vi "CmdCenter_SingleRecipe.vi"(8 "error in (no error)":errorcluster, 11 "Message_Queues":T2) -> (0 "error out":errorcluster)   [LabVIEW 2014]
uses:
  15_DataManagement/Config_RFSG.ctl
  02_Controls/Message_Queues.ctl
  02_Controls/Message_Data_Ctl.ctl
  15_DataManagement/Config_RFSA_IQ_Acq.ctl
  15_DataManagement/Config_RFSA_Spectrum_Acq.ctl
  15_DataManagement/Config_RFSA_Vertical.ctl
  <vilib>/Utility/file.llb/Read From Spreadsheet File (string).vi
panel:
  in  "Recipe_Index":i32
  in  "file path (dialog if empty)":path=path "C:/Gyuwon_Folder/SourceCodeFolder/1005_Gyu_RF_SourceProject_Msg/___SystemFiles/RecipeMode.ini"
  in  "Tab Control":enum32{"RFSG_Config"}(tab)
  out "Config_RFSG":T1={"Carrier Frequency"=1300000000.0, "RF Power Level (dBm)"=-20.0, "SG External Gain (dBm)"=0.0, "Standard"=enum."LTE"} {"SG External Gain (dBm)" format="%#_6p"; "RF Power Level (dBm)" format="%#_6p"; "Carrier Frequency" format="%#_6p"}
  in  "Update":bool
  in  "Stop Button":bool
  in  "Start":bool
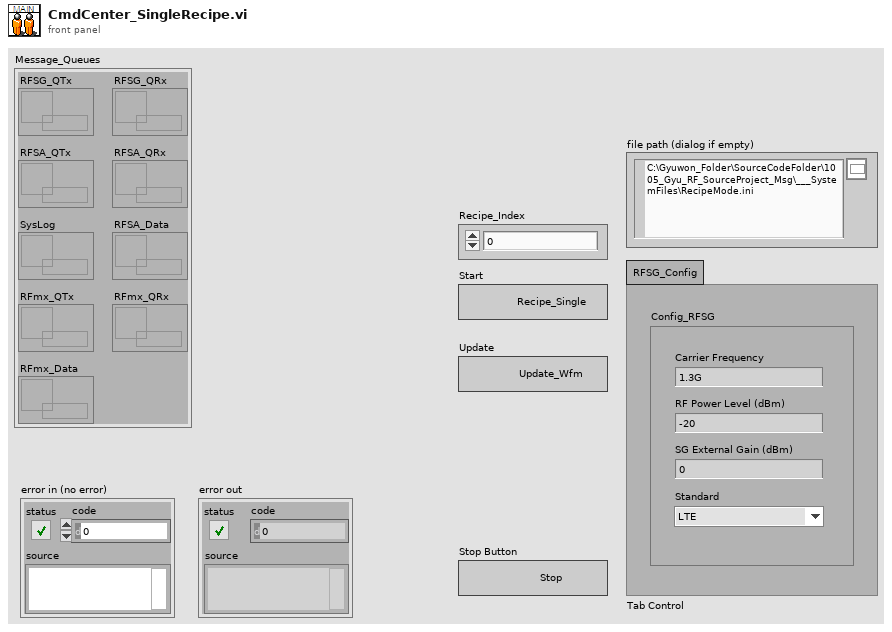
[diagram p1: front panel]
types:
  T1 = typedef "Config_RFSG.ctl" = cluster{"Carrier Frequency":dbl, "RF Power Level (dBm)":dbl, "SG External Gain (dBm)":dbl, "Standard":enum16{"LTE", "WCDMA", "GSM", "EDGE", "CW", "CWM"}}
  T2 = typedef "Message_Queues.ctl" = cluster{"RFSG_QTx":refnum<queue>, "RFSG_QRx":refnum<queue>, "RFSA_QTx":refnum<queue>, "RFSA_QRx":refnum<queue>, "SysLog":refnum<queue>, "RFSA_Data":refnum<queue>, "RFmx_QTx":refnum<queue>, "RFmx_QRx":refnum<queue>, "RFmx_Data":refnum<queue>}
  T3 = typedef "Config_RFSA_Vertical.ctl" = cluster{"Acquisition Type":i32, "Reference Level (dBm)":dbl, "External Gain (dB)":dbl}
  T4 = typedef "Config_RFSA_Spectrum_Acq.ctl" = cluster{"Resolution Bandwidth (Hz)":dbl, "Start Frequency (Hz)":dbl, "Stop Frequency (Hz)":dbl}
  T5 = typedef "Config_RFSA_IQ_Acq.ctl" = cluster{"carrier frequency":dbl, "IQ rate (S/s)":dbl, "samples per record":i64}
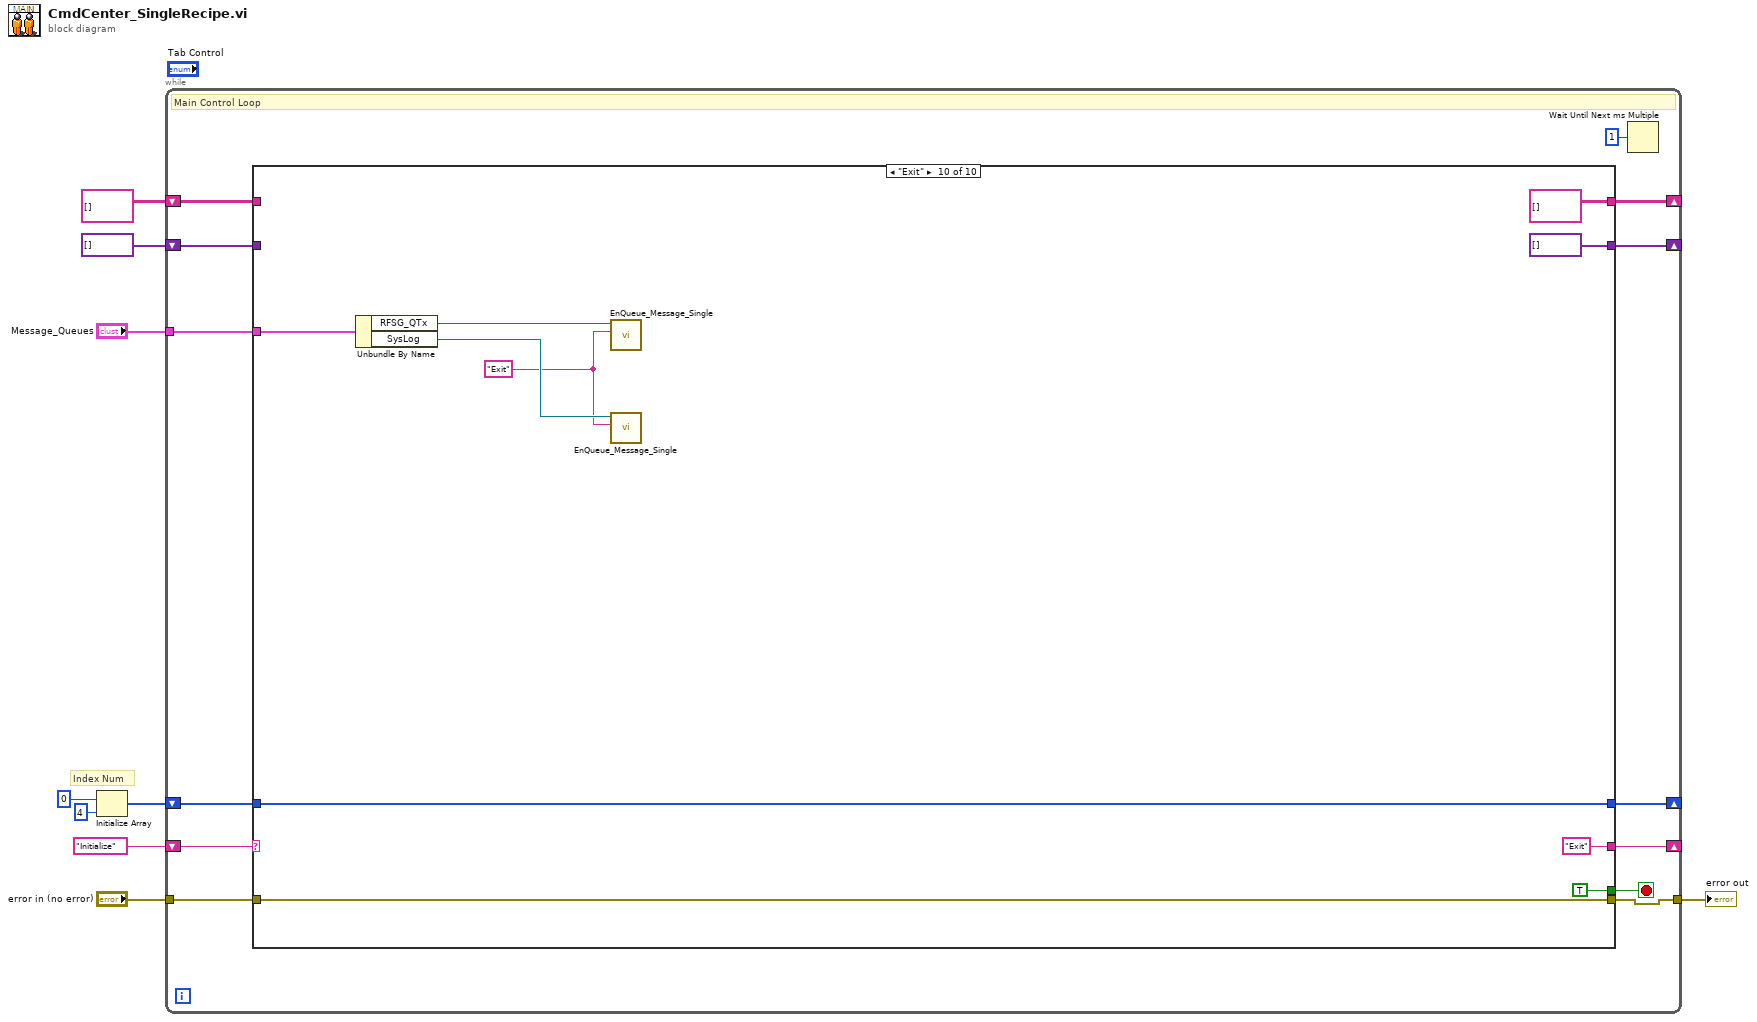
[diagram p0: block diagram]
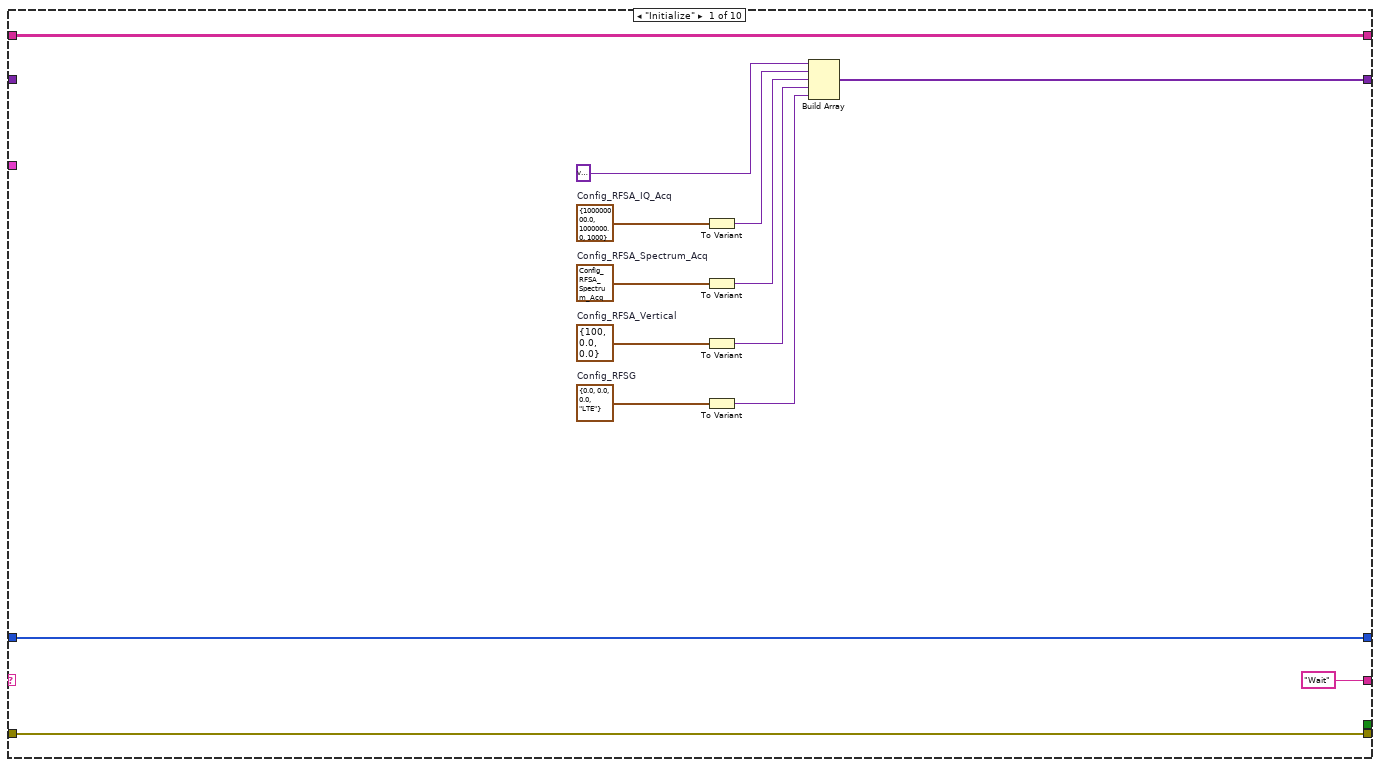
[diagram p2: hidden frame]
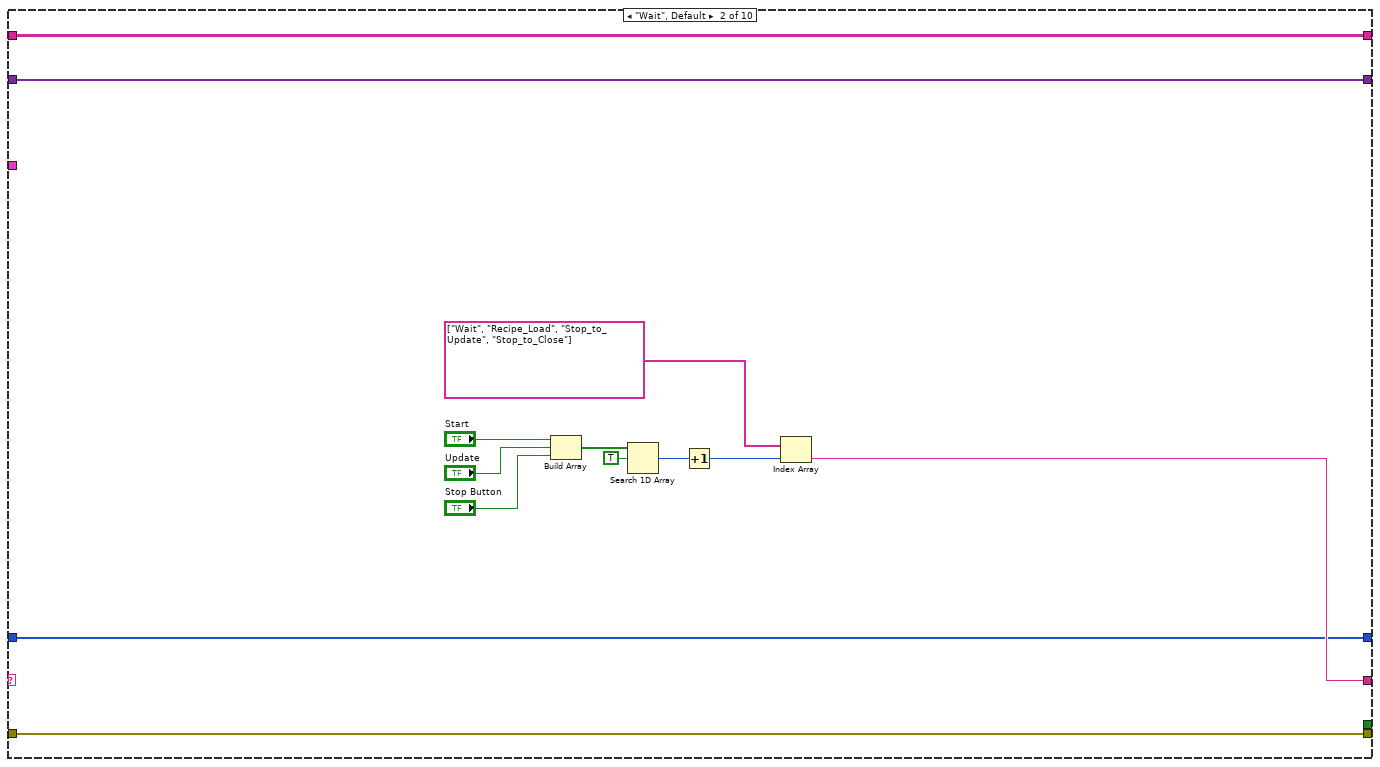
[diagram p3: hidden frame]
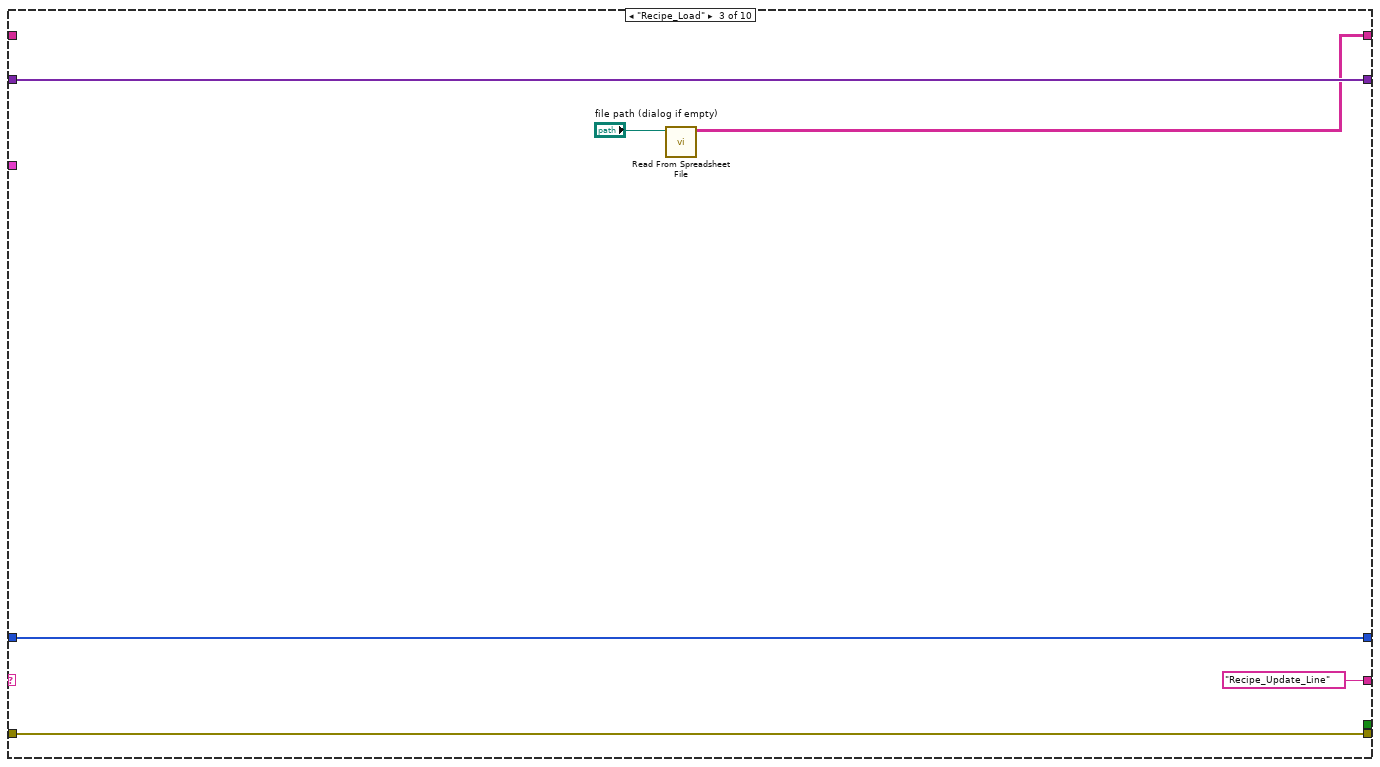
[diagram p4: hidden frame]
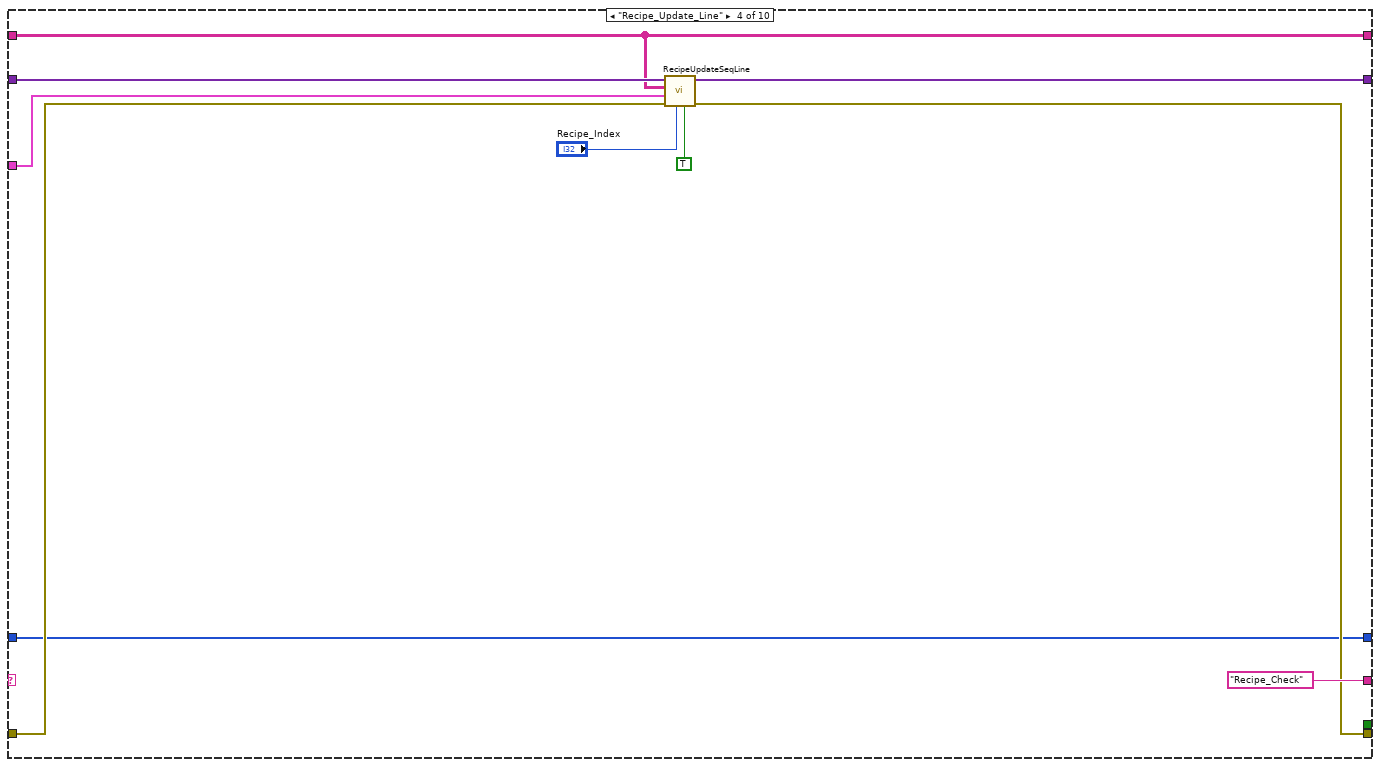
[diagram p5: hidden frame]
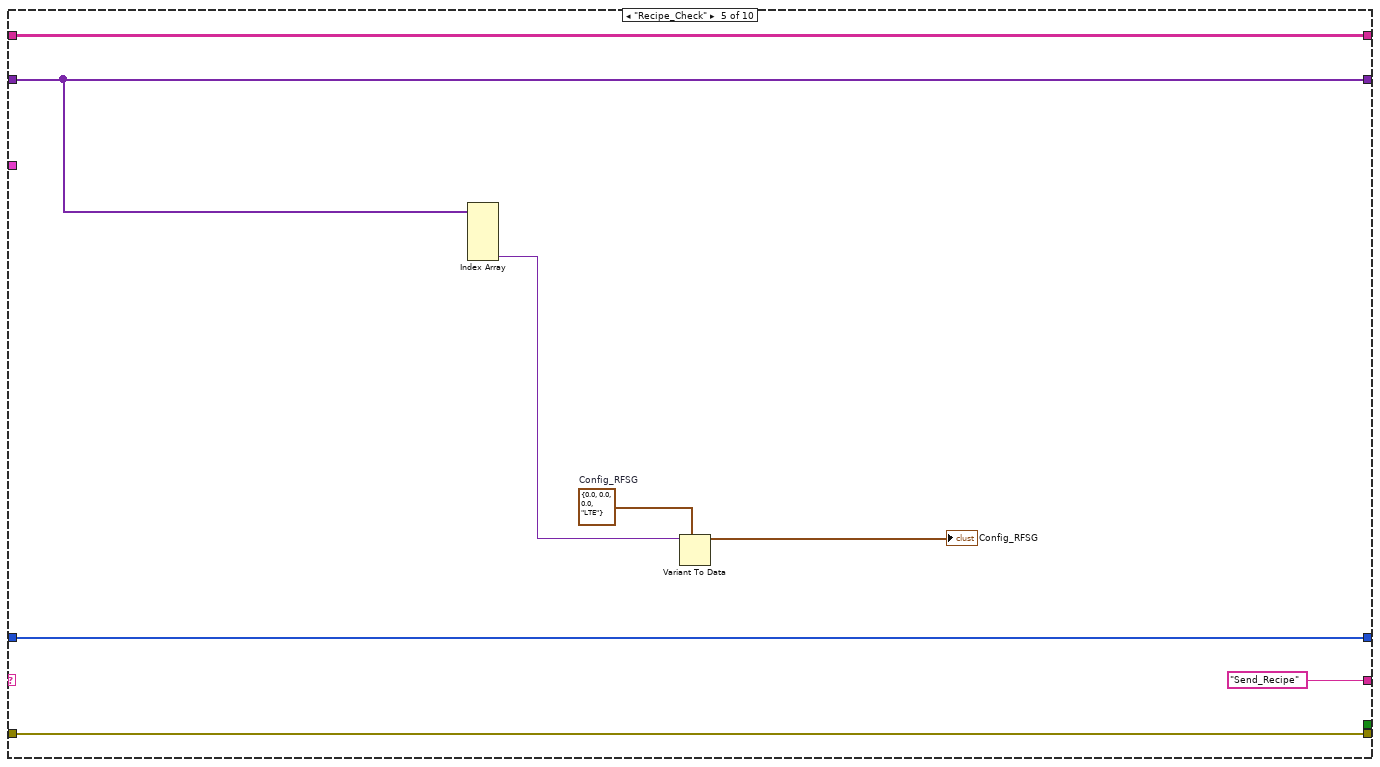
[diagram p6: hidden frame]
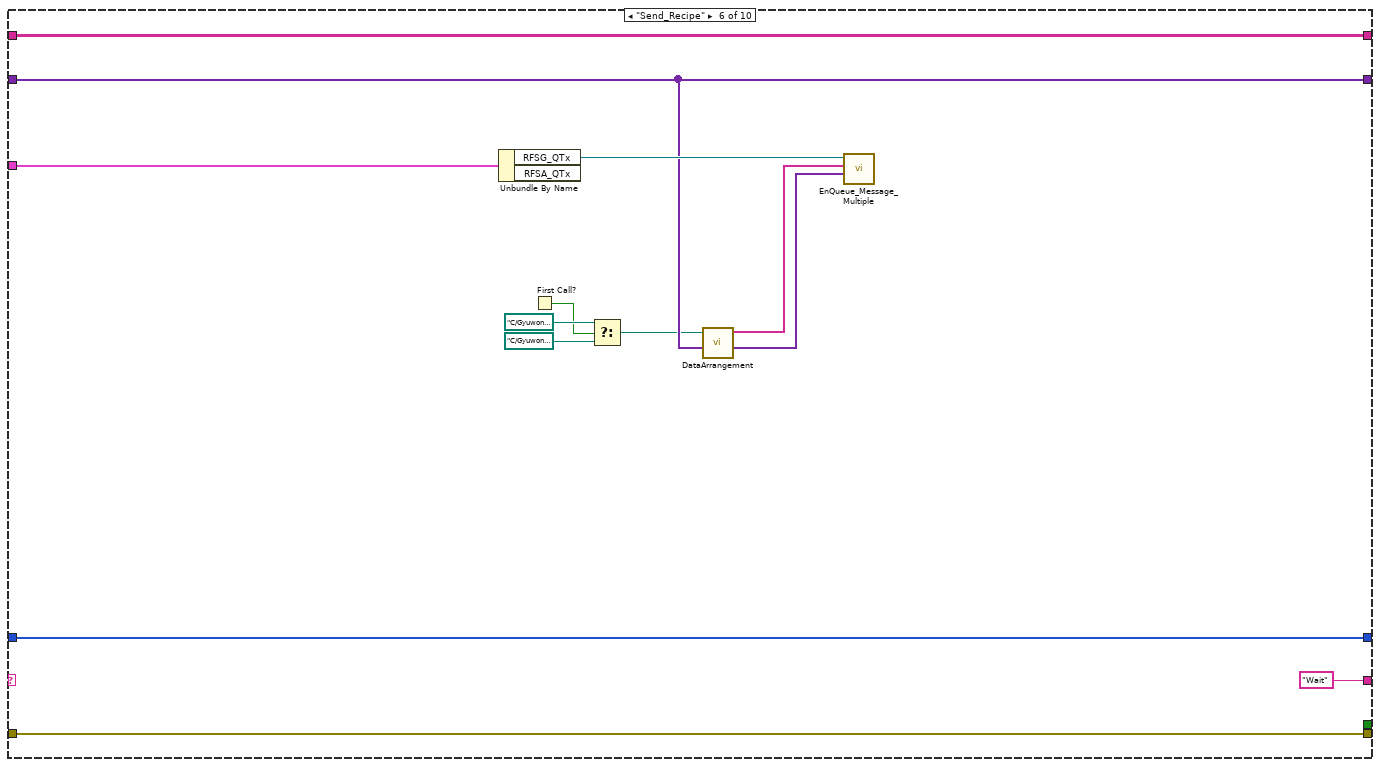
[diagram p7: hidden frame]
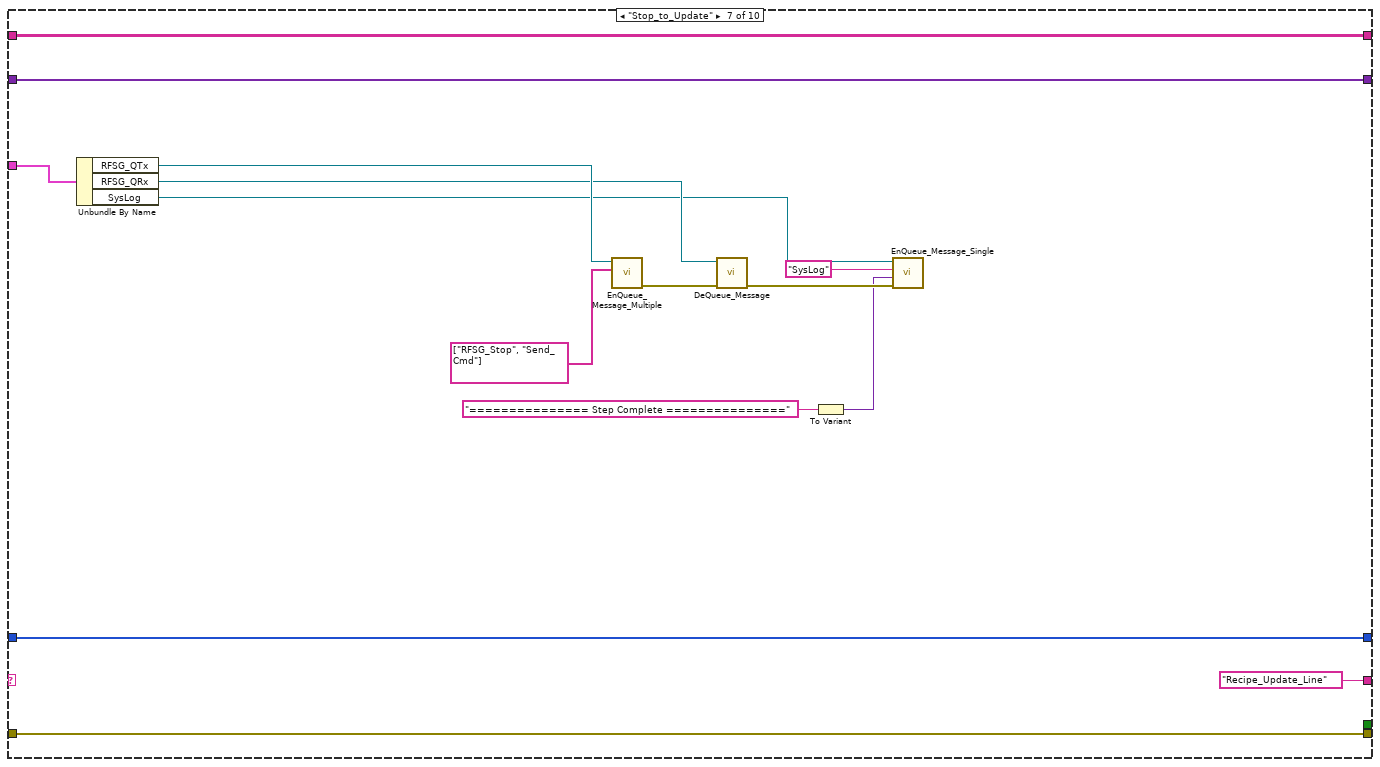
[diagram p8: hidden frame]
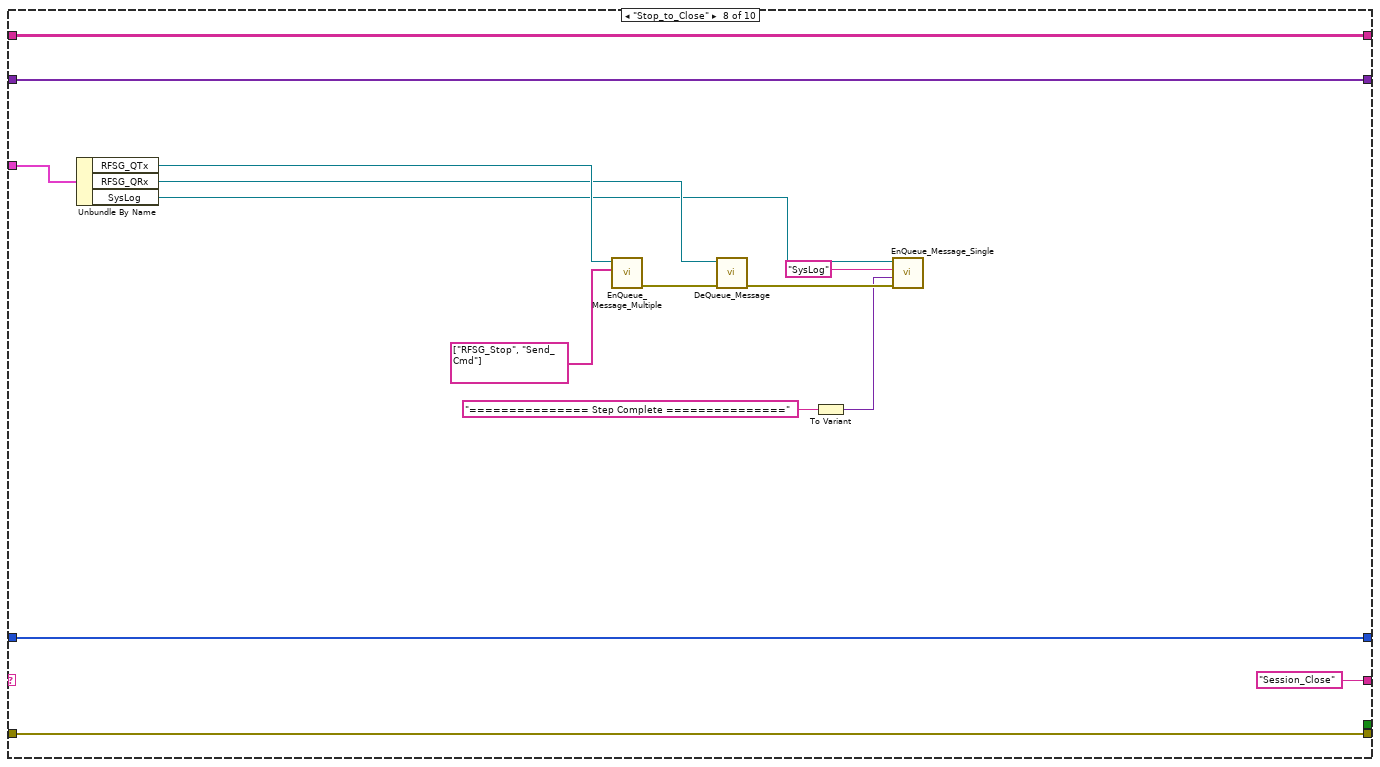
[diagram p9: hidden frame]
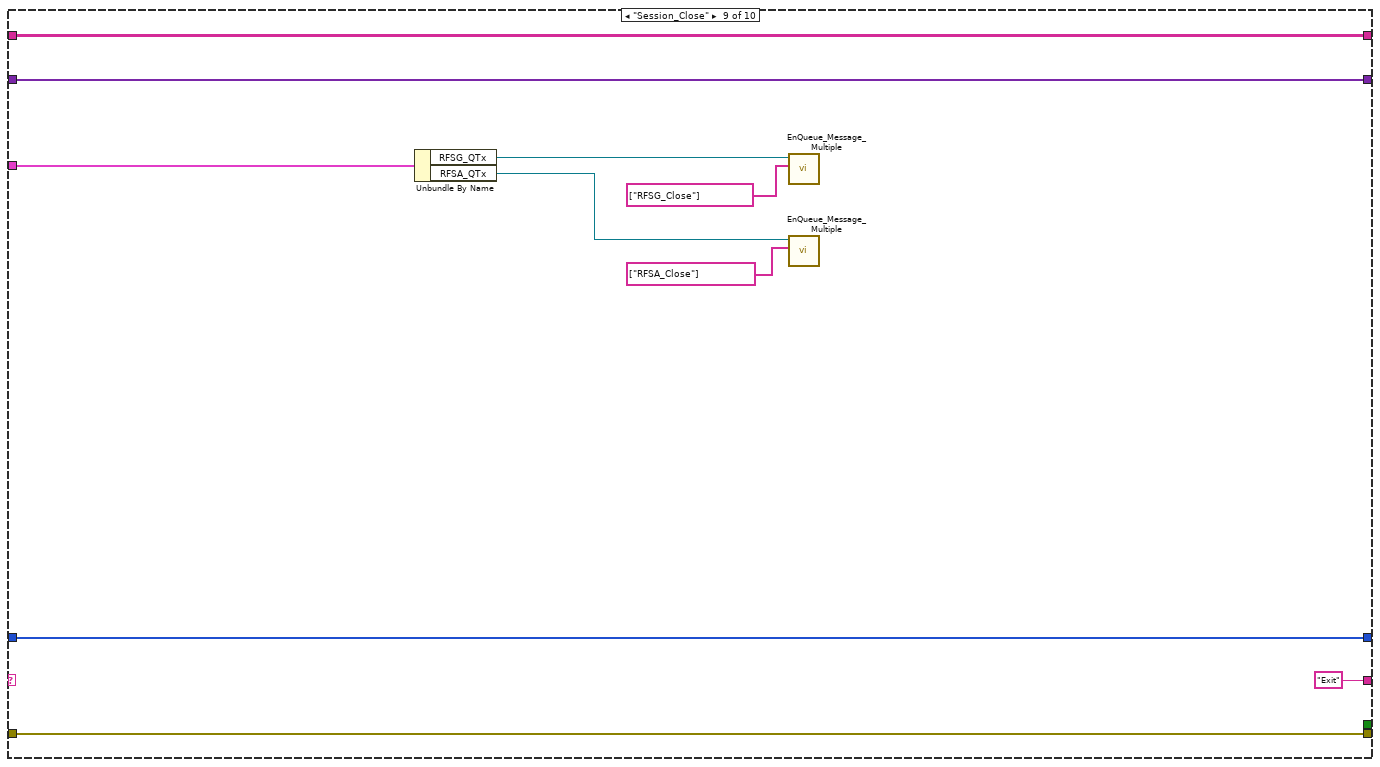
[diagram p10: hidden frame]
diagram:
  # "Index Num"
  n1 = Initialize Array(0, 4 ("dimension size")) -> (w1:i32[])
  n2 = while {
    tunnel: "error in (no error)" -> [w18]
    tunnel: [w21] -> w8
    tunnel: "Message_Queues" -> [w19]
    shift-right: [w16] -> _
    shift-left: "Initialize" -> [w20]
    shift-right: [w14] -> _
    shift-left: variant[] [] ("appended array") -> [w15]
    shift-right: [w13] -> _
    shift-left: string[][] [] ("all rows") -> [w12]
    shift-right: [w10] -> _
    shift-left: w1 -> [w11]
    stop <- w22 stop-if-true
    # "Main Control Loop"
    n3 = case shown="\"Exit\"" w20 {
      tunnel: w18 -> [w36 w49 w51 w62 w72 w86 w99 w114 w120 w135]
      tunnel: [_ _ _ _ _ _ _ _ _ TRUE] -> w22
      tunnel: [w36 w49 w51 w61 w72 w86 w99 w114 w120 w135] -> w21
      tunnel: w19 -> [_ _ _ w58 _ w85 w100 w115 w125 w133]
      tunnel: ["Wait" w40 "Recipe_Update_Line" "Recipe_Check" "Send_Recipe" "Wait" "Recipe_Update_Line" "Session_Close" "Exit" "Exit"] -> w16
      tunnel: w15 -> [_ w39 w55 w64 w71 w80 w98 w113 w119 _]
      tunnel: [w25 w39 w55 w63 w71 w80 w98 w113 w119 variant[] [] ("appended array")] -> w14
      tunnel: [w24 w38 w53 w60 w67 w79 w97 w112 w118 string[][] [] ("all rows")] -> w13
      tunnel: w12 -> [w24 w38 _ w60 w67 w79 w97 w112 w118 _]
      tunnel: w11 -> [w23 w37 w50 w59 w66 w78 w96 w111 w117 w127]
      tunnel: [w23 w37 w50 w59 w66 w78 w96 w111 w117 w127] -> w10
      frame "Initialize" {
        w33 = T1 {"Carrier Frequency"=0.0, "RF Power Level (dBm)"=0.0, "SG External Gain (dBm)"=0.0, "Standard"=enum."LTE"}  # Config_RFSG
        w32 = T3 {"Acquisition Type"=100, "Reference Level (dBm)"=0.0, "External Gain (dB)"=0.0}  # Config_RFSA_Vertical
        w31 = T4 {"Resolution Bandwidth (Hz)"=10000.0, "Start Frequency (Hz)"=90000000.0, "Stop Frequency (Hz)"=110000000.0}  # Config_RFSA_Spectrum_Acq
        w34 = T5 {"carrier frequency"=100000000.0, "IQ rate (S/s)"=1000000.0, "samples per record"=1000}  # Config_RFSA_IQ_Acq
        n4 = To Variant(anything=w34) -> (Variant=w29:variant)
        n5 = To Variant(anything=w31) -> (Variant=w28:variant)
        n6 = To Variant(anything=w32) -> (Variant=w27:variant)
        n7 = To Variant(anything=w33) -> (Variant=w26:variant)
        n8 = Build Array(variant, w29, w28, w27, w26) -> (w25:variant[])
      }
      frame "Wait", Default {
        n9 = Build Array("Start", "Update", "Stop Button") -> (w45:bool[])
        n10 = Search 1D Array(1D array=w45, element=TRUE) -> (index of element=w43:i32)  [unwired: 1 in]
        n11 = Increment(x=w43) -> (x+1=w42:i32)
        n12 = Index Array(array=string[] ["Wait", "Recipe_Load", "Stop_to_Update", "Stop_to_Close"], index=w42) -> (element=w40:string)
      }
      frame "Recipe_Load" {
        n13 = call-poly <vilib>:"Read From Spreadsheet File.vi"("file path (dialog if empty)"="file path (dialog if empty)") -> ("all rows"=w53:string[][])  [unwired: 6 in, 4 out]
      }
      frame "Recipe_Update_Line" {
        n14 = call "RecipeUpdateSeqLine.vi"("LogClear?"=TRUE, "Seq_Index"="Recipe_Index", "error in (no error)"=w62, "Message_Queues"=w58, "Recipe_Input"=w60, "DeviceSetup"=w64) -> ("error out"=w61:errorcluster, "DeviceSetup_Update"=w63:variant[])  [unwired: 4 in]
      }
      frame "Recipe_Check" {
        w70 = T1 {"Carrier Frequency"=0.0, "RF Power Level (dBm)"=0.0, "SG External Gain (dBm)"=0.0, "Standard"=enum."LTE"}  # Config_RFSG
        n15 = Index Array(array=w71) -> (element #5=w69:variant)  [unwired: 5 in, 4 out]
        n16 = Variant To Data(type=w70, Variant=w69) -> (data=→"Config_RFSG":T1)  [unwired: 1 in, 1 out]
      }
      frame "Send_Recipe" {
        n17 = Unbundle By Name(w85) -> ("RFSG_QTx"=w84:refnum<queue>)  [unwired: 1 out]
        n18 = First Call?() -> (First Call?: T/F=w75:bool)
        n19 = Select(t=path "C:/Gyuwon_Folder/SourceCodeFolder/1005_Gyu_RF_SourceProject_Msg/___SystemFiles/RFSG_Default_Setting.csv" ("RFSG_List_1st"), s=w75, f=path "C:/Gyuwon_Folder/SourceCodeFolder/1005_Gyu_RF_SourceProject_Msg/___SystemFiles/RFSG_Change_Setting.csv" ("RFSG_List_1st")) -> (s? t:f=w74:path)
        n20 = call "DataArrangement.vi"("DataType"=w80, "file path (dialog if empty)"=w74) -> ("DataList"=w81:variant[], "CmdList"=w82:string[])  [unwired: 7 in, 1 out]
        n21 = call "EnQueue_Message_Multiple.vi"("Message Data Array"=w81, "Message Array"=w82, "Message_Queue"=w84) -> ()  [unwired: 7 in, 2 out]
      }
      frame "Stop_to_Update" {
        n22 = Unbundle By Name(w100) -> ("RFSG_QTx"=w94:refnum<queue>, "RFSG_QRx"=w92:refnum<queue>, "SysLog"=w90:refnum<queue>)
        n23 = call "EnQueue_Message_Multiple.vi"("Message Array"=string[] ["RFSG_Stop", "Send_Cmd"], "Message_Queue"=w94) -> ("error out"=w93:errorcluster)  [unwired: 8 in, 1 out]
        n24 = call "DeQueue_Message.vi"("error in (no error)"=w93, "Message_Queue"=w92) -> ("error out"=w91:errorcluster)  [unwired: 6 in, 3 out]
        n25 = To Variant(anything="=============== Step Complete ===============" ("Message")) -> (Variant=w87:variant)
        n26 = call "EnQueue_Message_Single.vi"("error in (no error)"=w91, "Message Data"=w87, "Message"="SysLog", "Message_Queue"=w90) -> ()  [unwired: 6 in, 2 out]
      }
      frame "Stop_to_Close" {
        n27 = Unbundle By Name(w115) -> ("RFSG_QTx"=w109:refnum<queue>, "RFSG_QRx"=w107:refnum<queue>, "SysLog"=w105:refnum<queue>)
        n28 = call "EnQueue_Message_Multiple.vi"("Message Array"=string[] ["RFSG_Stop", "Send_Cmd"], "Message_Queue"=w109) -> ("error out"=w108:errorcluster)  [unwired: 8 in, 1 out]
        n29 = call "DeQueue_Message.vi"("error in (no error)"=w108, "Message_Queue"=w107) -> ("error out"=w106:errorcluster)  [unwired: 6 in, 3 out]
        n30 = To Variant(anything="=============== Step Complete ===============" ("Message")) -> (Variant=w102:variant)
        n31 = call "EnQueue_Message_Single.vi"("error in (no error)"=w106, "Message Data"=w102, "Message"="SysLog", "Message_Queue"=w105) -> ()  [unwired: 6 in, 2 out]
      }
      frame "Session_Close" {
        n32 = Unbundle By Name(w125) -> ("RFSG_QTx"=w124:refnum<queue>, "RFSA_QTx"=w122:refnum<queue>)
        n33 = call "EnQueue_Message_Multiple.vi"("Message Array"=string[] ["RFSG_Close"], "Message_Queue"=w124) -> ()  [unwired: 8 in, 2 out]
        n34 = call "EnQueue_Message_Multiple.vi"("Message Array"=string[] ["RFSA_Close"], "Message_Queue"=w122) -> ()  [unwired: 8 in, 2 out]
      }
      frame "Exit" {
        w130 = "Exit" ("Message")
        n35 = Unbundle By Name(w133) -> ("RFSG_QTx"=w132:refnum<queue>, "SysLog"=w131:refnum<queue>)
        n36 = call "EnQueue_Message_Single.vi"("Message"=w130, "Message_Queue"=w132) -> ()  [unwired: 8 in, 2 out]
        n37 = call "EnQueue_Message_Single.vi"("Message"=w130, "Message_Queue"=w131) -> ()  [unwired: 8 in, 2 out]
      }
    }
    n38 = Wait Until Next ms Multiple(millisecond multiple=u32 1) -> ()  [unwired: 1 out]
  }
  "error out" <- w8
